vi "Main.vi"(11 "Module Admin":refnum<class "Delacor_lib_QMH_Module Admin.lvclass">) -> ()   [LabVIEW 2021, in "Test Panel GUI Update.lvlib"]
doc: "This template is based off of the Queued Message Handler design pattern and the Queued Message Handler project template that ships with LabVIEW.\n\nThe main difference is that the queue is private to this module and communication between modules is performed via Broadcast and Request events.\n\nRequest events are wrapped in public API methods and are handled in the Event Handling Loop (EHL) of this VI. Any module can register for Broadcast events sent by this module. The EHL generates messages based on user interface actions.\n\nThe Message Handling Loop (MHL) processes messages generated by the EHL, or by other messages. The messages are string values, so new messages can be added easily to the Message Cases case structure in the MHL. Each message cluster can also provide an optional value for Message Data, which is a variant that can be converted to whatever message-specific data is required.\n_____\nBased on DQMH Project Template 7.0.1.1316."
uses:
  Test Panel GUI Update.lvlib
  <vilib>/Delacor/Delacor QMH/Libraries/Module Admin_class/Delacor_lib_QMH_Module Admin.lvclass
  Module Data--cluster.ctl
  Test Panel/GUI Ctrl Data's--Cluster.ctl
  Test Panel/Rx-Mapping Data.ctl
  Capsule-Data's.ctl
  Host-Control's/DIO Data's from RT.ctl
  Host-Control's/AI-Data from RT.ctl
  <vilib>/Wovalab/Utilities/Helper Loop Periodic Timing/Helper Loop Periodic Timing.lvclass/Helper Loop Periodic Timing.ctl
  <vilib>/Delacor/Delacor QMH/Libraries/Message Queue_class/Delacor_lib_QMH_Message Queue.lvclass/Delacor_lib_QMH_Message Queue.ctl
  Host-Control's/Module ID Action Enum.ctl
  RT-Encode Data.ctl
  Stop Argument--cluster.ctl
  <vilib>/Delacor/Delacor QMH/Libraries/Module Admin_class/Delacor_lib_QMH_Module Admin.lvclass/Delacor_lib_QMH_Module Admin.ctl
  Get GUI Ctrl Data Argument--cluster.ctl
  Get GUI Mapping Data's Argument--cluster.ctl
  <vilib>/Utility/miscctls.llb/LVPointTypeDef.ctl
  <vilib>/Delacor/Delacor QMH/Libraries/Message Queue_class/Delacor_lib_QMH_Enqueue Message (Single).vi
  <vilib>/Delacor/Delacor QMH/Libraries/Module Admin_class/Delacor_lib_QMH_Get External Launch.vi
  <vilib>/Wovalab/Utilities/Helper Loop Periodic Timing/U32 Max Value--constant.vi
  <vilib>/Wovalab/Utilities/Helper Loop Periodic Timing/Update Last Execution Time.vi
  <vilib>/Wovalab/Utilities/Helper Loop Periodic Timing/Helper Loop Periodic Timing.lvclass
  <vilib>/Delacor/Delacor QMH/Libraries/Message Queue_class/Delacor_lib_QMH_Message Queue.lvclass
  Test Panel/Test Panel.lvlib
  RT Acquisition Engine/RT Acquisition Engine.lvlib
panel:
  out "error out":errorcluster
  out "Status":string
  in  "Simulate MHL Error":bool
  in  "Simulate EHL Error":bool
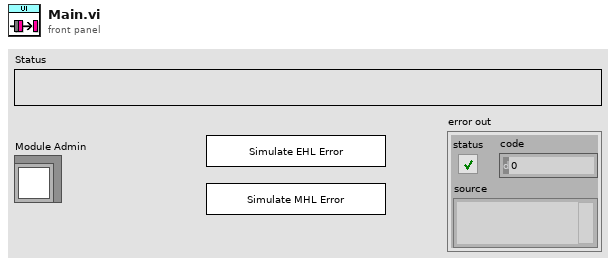
[diagram p1: front panel]
types:
  T1 = typedef "Test Panel GUI Update.lvlib/Request Events--cluster.ctl" = cluster{"Stop Module":refnum<user-event>, "Show Panel":refnum<user-event>, "Hide Panel":refnum<user-event>, "Get Module Execution Status":refnum<user-event>, "Show Diagram":refnum<user-event>, "Get GUI Ctrl Data":refnum<user-event>, "Get GUI Mapping Data's":refnum<user-event>}
  T2 = typedef "Test Panel GUI Update.lvlib/Module Data--cluster.ctl" = cluster{"Status":string, "GUI Ctrl Data's":T3, "Rx-Mapping Data":T4, "Capsule-Data's":T5, "AI Data's":map{string, dbl}}
  T3 = typedef "Test Panel.lvlib/GUI Ctrl Data's--Cluster.ctl" = cluster{"All Ctrl and Indi Label":string[], "All Ctrl & Indi Ref":refnum<vi>[]}
  T4 = typedef "Test Panel.lvlib/Rx-Mapping Data.ctl" = cluster{"Mapped Ctrl and Indi Label":string[], "Mapped Hardware Name":string[], "Mapped Interface Name":string[], "Mapped Channel Name":string[]}
  T5 = typedef "Test Panel GUI Update.lvlib/Capsule-Data's.ctl" = cluster{"DIO Data's":T6, "AI-Info":T7}
  T6 = typedef "DIO Data's from RT.ctl" = cluster{"Channels":string[], "Data":bool[], "Time":string}
  T7 = typedef "AI-Data from RT.ctl" = cluster{"Channel Name's":string[], "Channel Data's":dbl[], "Date & Time":string}
  T8 = typedef "Test Panel GUI Update.lvlib/RT-Encode Data.ctl" = cluster{"Hardware Name":string, "Interface Name":string, "Data":variant}
  T9 = typedef "Module ID Action Enum.ctl" = enum16{"Init", "Insert", "Get a ID", "Get all ID"}
  T10 = enum32{"invalid lock state", "Not Locked", "Locked (No Password)", "Password-protected"}
  T11 = typedef "Test Panel GUI Update.lvlib/Stop Argument--cluster.ctl" = cluster{"Origin":string, "Exit via Stop Module Req?":bool, "Wait for Module to stop?":bool}
  T12 = typedef "Test Panel GUI Update.lvlib/Get GUI Ctrl Data Argument--cluster.ctl" = cluster{"GUI Ctrl Data's":variant}
  T13 = typedef "Test Panel GUI Update.lvlib/Get GUI Mapping Data's Argument--cluster.ctl" = cluster{"Mapping Deatils":variant}
  T14 = typedef "LVPointTypeDef.ctl" = cluster{"Horizontal":i16, "Vertical":i16}
  T15 = enum32{"Invalid", "Standard", "Closed", "Hidden", "Minimized", "Maximized"}
  T16 = typedef "RT Acquisition Engine.lvlib/Broadcast Events--cluster.ctl" = cluster{"Module Did Init":refnum<user-event>, "Status Updated":refnum<user-event>, "Error Reported":refnum<user-event>, "Module Did Stop":refnum<user-event>, "Update Module Execution Status":refnum<user-event>, "RT Connection Status":refnum<user-event>, "Tx RT Hardware Info":refnum<user-event>, "DO Data's":refnum<user-event>, "AI-Info":refnum<user-event>}
  T17 = typedef "HW Name Enum.ctl" = enum16{"Capsule-1", "Capsule-2", "Capsule-3", "Capsule-4", "sb-RIO", "Safety", "Release"}
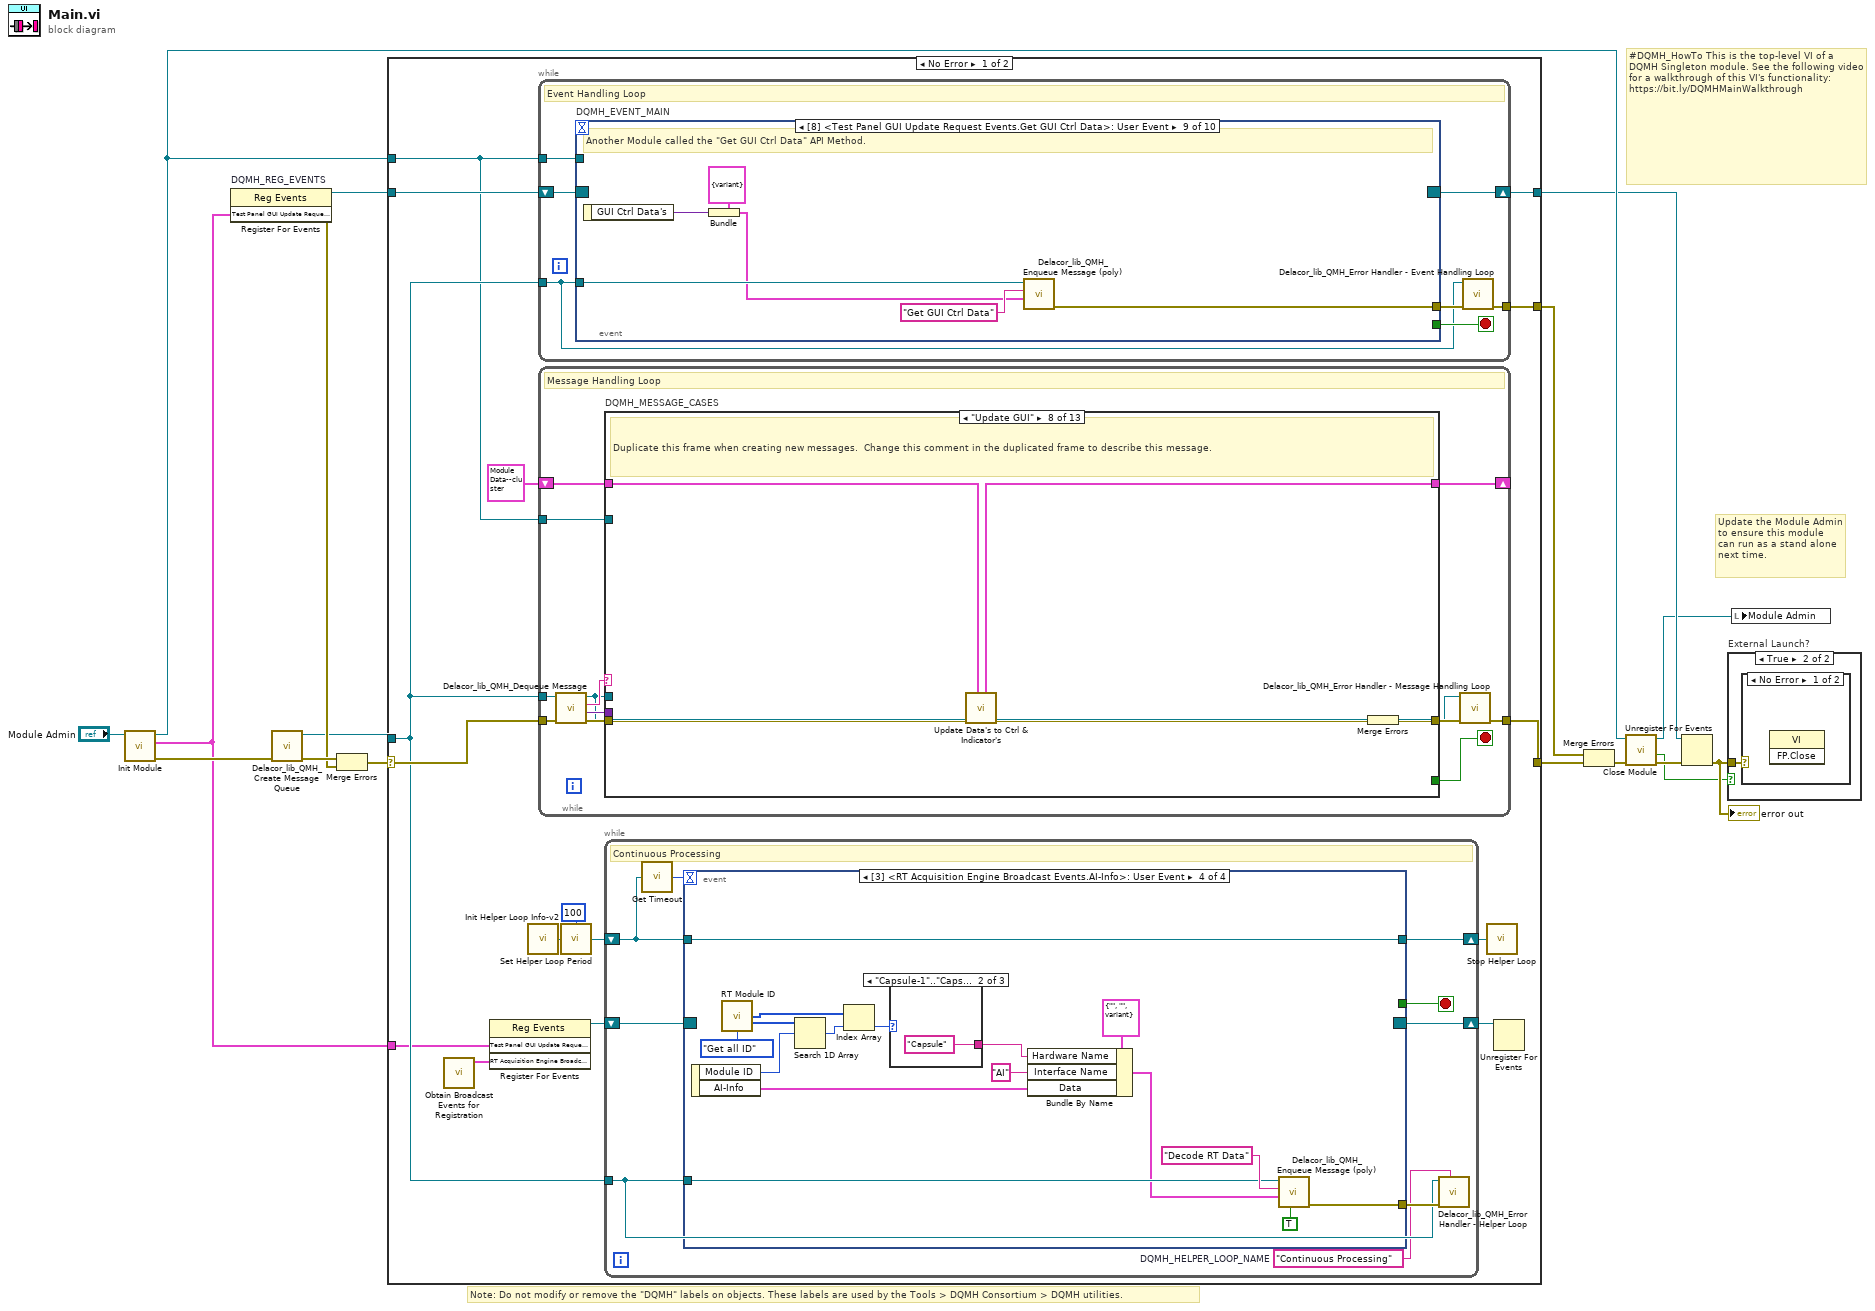
[diagram p0: block diagram]
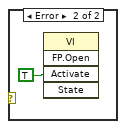
[diagram p3: hidden frame]
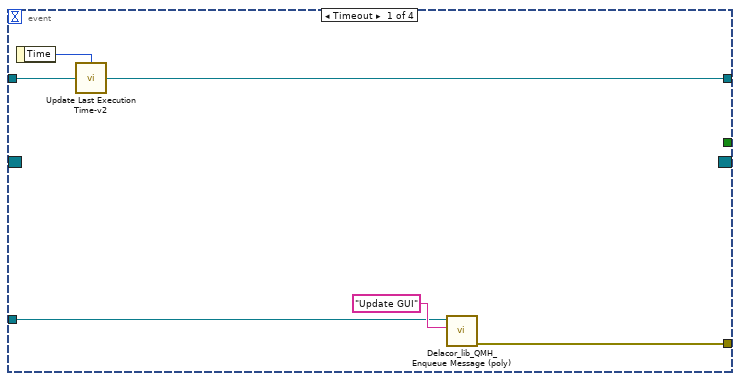
[diagram p4: hidden frame]
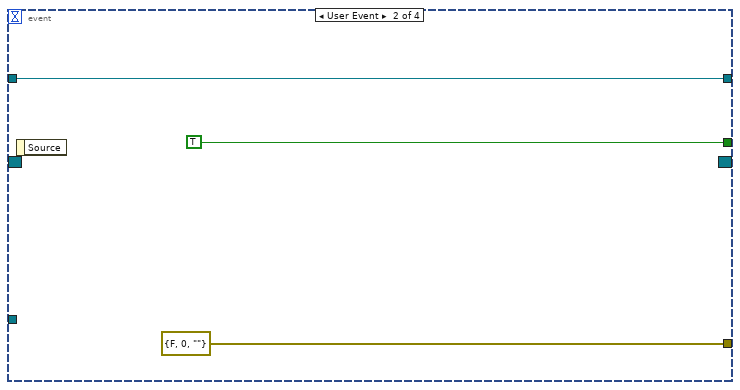
[diagram p5: hidden frame]
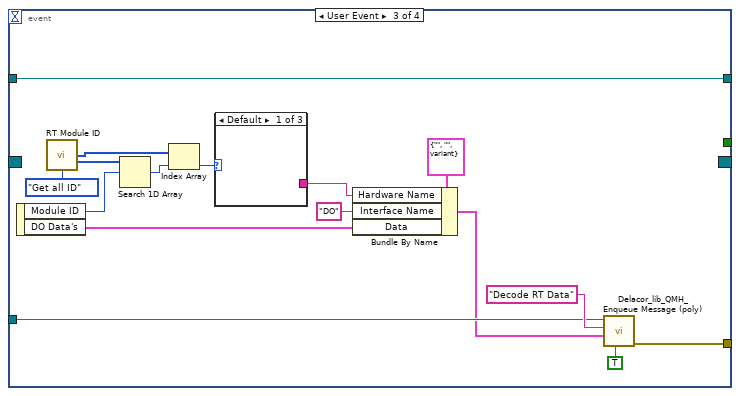
[diagram p6: hidden frame]
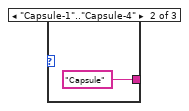
[diagram p7: hidden frame]
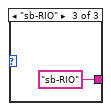
[diagram p8: hidden frame]
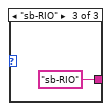
[diagram p10: hidden frame]
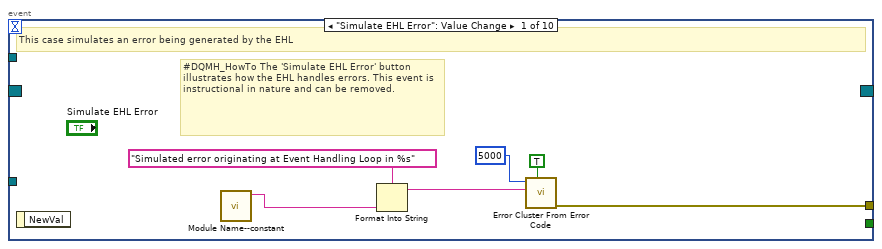
[diagram p11: hidden frame]
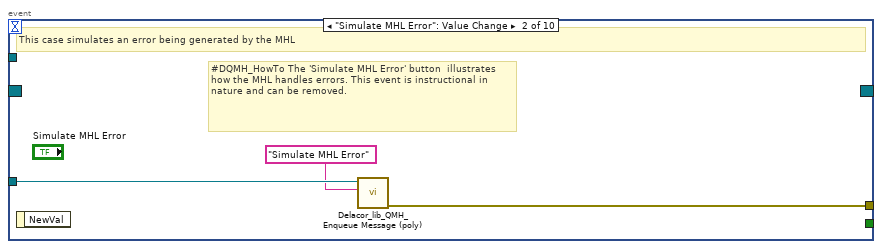
[diagram p12: hidden frame]
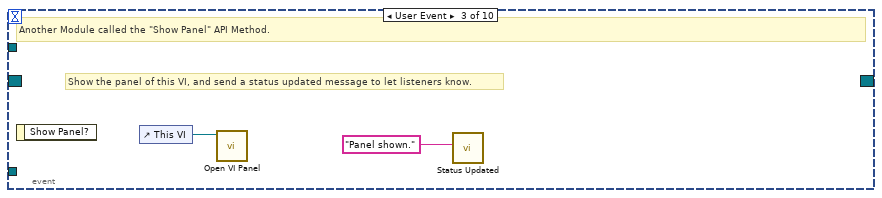
[diagram p13: hidden frame]
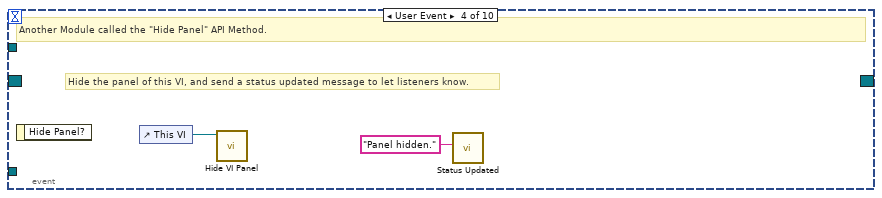
[diagram p14: hidden frame]
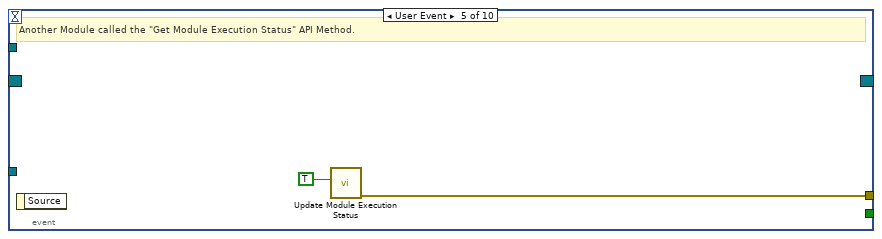
[diagram p15: hidden frame]
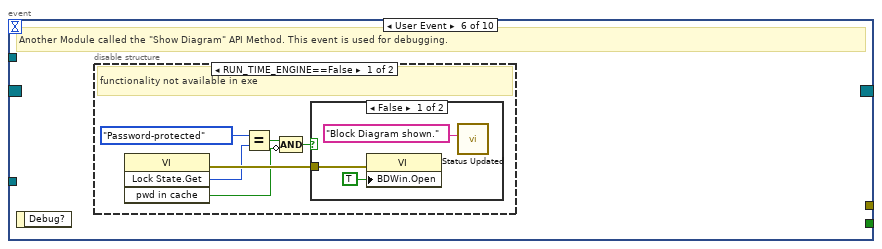
[diagram p16: hidden frame]
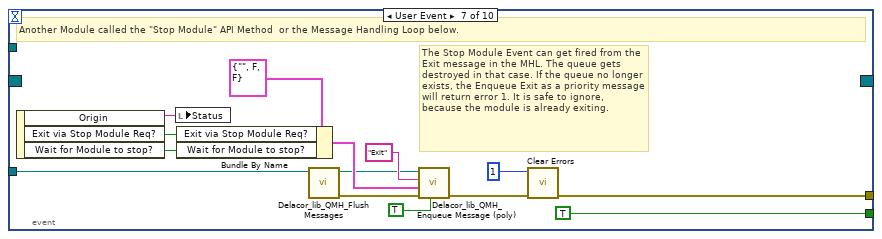
[diagram p19: hidden frame]
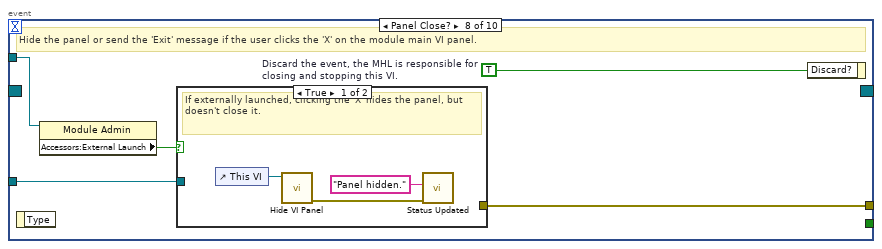
[diagram p20: hidden frame]
diagram:
  # "#DQMH_HowTo This is the top-level VI of a DQMH Singleton module. See the following video for a walkthrough of this VI's functionality: https://bit.ly/DQMHMainWalkthrough"
  # "Note: Do not modify or remove the \"DQMH\" labels on objects. These labels are used by the Tools > DQMH Consortium > DQMH utilities."
  # "Update the Module Admin to ensure this module can run as a stand alone next time."
  n1 = call "Init Module.vi"("Singleton Module Admin in"="Module Admin") -> ("error out"=w16:errorcluster, "Test Panel GUI Update Request Events"=w1:T1, "Singleton Module Admin out"=w8:refnum<class "Delacor_lib_QMH_Module Admin.lvclass">)  [unwired: 8 in]
  n2 = register-events "DQMH_REG_EVENTS"(w1) -> (reference out=w6:refnum<event-registration>, error out=w9:errorcluster)  [unwired: 2 in]
  n3 = call <vilib>:"Delacor_lib_QMH_Create Message Queue.vi"("error in"=w16) -> ("error out"=w11:errorcluster, "Message Queue"=w5:refnum<class "Delacor_lib_QMH_Message Queue.lvclass">)  [unwired: 9 in]
  n4 = Merge Errors(w11, w9) -> (w10:errorcluster)
  n5 = case shown="No Error" w10 {
    selector: w10 -> [w31 w296]
    tunnel: [w33 w295] -> w17
    tunnel: [w30 w294] -> w7
    tunnel: w6 -> [w28 w294]
    tunnel: w5 -> [w27 w289]
    tunnel: [w32 _] -> w14
    tunnel: w8 -> [w26 w290]
    tunnel: w1 -> [w25 _]
    frame No Error {
      n6 = call "Obtain Broadcast Events for Registration.vi"() -> ("RT Acquisition Engine Broadcast Events"=w18:T16)  [unwired: 9 in, 2 out]
      n7 = register-events ("DQMH_HELPER_REGFOREVENTS")(w25, w18) -> (reference out=w23:refnum<event-registration>)  [unwired: 2 in, 1 out]
      n8 = call <vilib>:"Init Helper Loop Info-v2.vi"() -> ("Helper Loop Periodic Timing"=w20:refnum<class "Helper Loop Periodic Timing.lvclass">)  [unwired: 1 in]
      n9 = while {
        tunnel: w27 -> [w88]
        shift-right: [w91] -> w30
        shift-left: w28 -> [w92]
        tunnel: [w93] -> w32
        tunnel: w26 -> [w89]
        stop <- w90 stop-if-true
        # "Event Handling Loop"
        n10 = event "DQMH_EVENT_MAIN" shown="[8] <Test Panel GUI Update Request Events.Get GUI Ctrl Data>: User Event" {
          selector: w92 -> [_ _ _ _ _ _ _ _ _ _]
          dyn-events: [_ _ _ _ _ _ _ _ _ _] -> w91
          timeout: _ -> [_ _ _ _ _ _ _ _ _ _]
          tunnel: [_ _ _ _ _ _ TRUE ("Discard?") _ _ _] -> w90
          tunnel: w88 -> [_ w102 _ _ _ _ w121 w135 w150 w156]
          tunnel: [w100 w103 _ _ w109 _ w131 w137 w145 w151] -> w94
          tunnel: w89 -> [_ _ _ _ _ _ _ w134 _ _]
          event "Simulate EHL Error": Value Change {
            # "#DQMH_HowTo The 'Simulate EHL Error' button  illustrates how the EHL handles errors. This event is instructional in nature and can be removed."
            # "This case simulates an error being generated by the EHL"
            n11 = event-data() -> ()  [unwired: 1 in, 1 out]
            n12 = call "Module Name--constant.vi"() -> ("Module Name"=w97:string)  [unwired: 11 in]
            n13 = Format Into String(format string="Simulated error originating at Event Handling Loop in %s", w97) -> (resulting string=w98:string)  [unwired: 2 in, 1 out]
            n14 = call <vilib>:"Error Cluster From Error Code.vi"("show call chain? (False)"=TRUE, "error message (\"\")"=w98, "error code (0)"=5000) -> ("error out"=w100:errorcluster)  [unwired: 6 in]
          }
          event "Simulate MHL Error": Value Change {
            # "#DQMH_HowTo The 'Simulate MHL Error' button  illustrates how the MHL handles errors. This event is instructional in nature and can be removed."
            # "This case simulates an error being generated by the MHL"
            n15 = event-data() -> ()  [unwired: 1 in, 1 out]
            n16 = call-poly <vilib>:"Delacor_lib_QMH_Enqueue Message (poly).vi"("Message"="Simulate MHL Error", "Message Queue in"=w102) -> ("error out"=w103:errorcluster)  [unwired: 8 in, 1 out]
          }
          event User Event {
            # "Show the panel of this VI, and send a status updated message to let listeners know."
            # "Another Module called the \"Show Panel\" API Method."
            n17 = event-data() -> ()  [unwired: 1 in, 1 out]
            n18 = control-ref of="This VI"() -> (w105:refnum<vi>)
            n19 = call "Open VI Panel.vi"("VI"=w105) -> ()  [unwired: 10 in, 1 out]
            n20 = call "Status Updated.vi"("Status"="Panel shown." ("format string")) -> ()  [unwired: 10 in, 1 out]
          }
          event User Event {
            # "Hide the panel of this VI, and send a status updated message to let listeners know."
            # "Another Module called the \"Hide Panel\" API Method."
            n21 = event-data() -> ()  [unwired: 1 in, 1 out]
            n22 = control-ref of="This VI"() -> (w107:refnum<vi>)
            n23 = call "Hide VI Panel.vi"("VI"=w107) -> ()  [unwired: 10 in, 1 out]
            n24 = call "Status Updated.vi"("Status"="Panel hidden." ("format string")) -> ()  [unwired: 10 in, 1 out]
          }
          event User Event {
            # "Another Module called the \"Get Module Execution Status\" API Method."
            n25 = event-data() -> ()  [unwired: 1 in, 1 out]
            n26 = call "Update Module Execution Status.vi"("Running?"=TRUE) -> ("error out"=w109:errorcluster)  [unwired: 10 in]
          }
          event User Event {
            # "Another Module called the \"Show Diagram\" API Method. This event is used for debugging."
            n27 = event-data() -> ()  [unwired: 1 in, 1 out]
            n28 = disable-structure shown="RUN_TIME_ENGINE==False" {
              frame condition #0 (active) {
                # "functionality not available in exe"
                n29 = invoke on="Invoke Node" class="VI" method="Lock State.Get"() -> (error out=w115:errorcluster, "Get Lock State"=w114:T10, "pwd in cache"=w111:bool)  [unwired: 4 in, 1 out]
                n30 = Equal?(x=T10."Password-protected", y=w114) -> (x = y?=w112:bool)
                n31 = Compound Arithmetic op=AND(w112, invert w111) -> (w110:bool)
                n32 = case shown="False" w110 {
                  tunnel: w115 -> [w118 _]
                  frame False {
                    n33 = property on="Property Node" class="VI"(error in=w118, "BDWin.Open"=TRUE ("Block Diagram Window:Open")) -> ()  [unwired: 1 in, 2 out]
                    n34 = call "Status Updated.vi"("Status"="Block Diagram shown." ("format string")) -> ()  [unwired: 10 in, 1 out]
                  }
                  frame True {
                    # "Password-protected VI, and the password is not in the cache. Do not show the diagram."
                  }
                }
              }
              frame condition #1 {
              }
            }
          }
          event User Event {
            # "The Stop Module Event can get fired from the Exit message in the MHL. The queue gets destroyed in that case. If the queue no longer exists, the Enqueue Exit as a priority message will return error 1. It is safe to ignore, because the module is already exiting."
            # "Another Module called the \"Stop Module\" API Method  or the Message Handling Loop below."
            n35 = event-data() -> ("Origin"=w128:string, "Exit via Stop Module Req?"=w124:bool, "Wait for Module to stop?"=w123:bool)  [unwired: 1 in]
            n36 = local write "Status"(w128) -> ()
            n37 = Bundle By Name(cluster=T11 {"Origin"="", "Exit via Stop Module Req?"=FALSE, "Wait for Module to stop?"=FALSE} ("Stop Argument"), "Exit via Stop Module Req?"=w124, "Wait for Module to stop?"=w123) -> (w122:T11)
            n38 = call-dynamic "Delacor_lib_QMH_Flush Messages.vi"("Message Queue in"=w121) -> ("error out"=w119:errorcluster, "Message Queue out"=w120:refnum<class "Delacor_lib_QMH_Message Queue.lvclass">)  [unwired: 7 in, 2 out]
            n39 = call-poly <vilib>:"Delacor_lib_QMH_Enqueue Message (poly).vi"("Priority Message? (F)"=TRUE, "error in"=w119, "Message Data"=w122, "Message"="Exit", "Message Queue in"=w120) -> ("error out"=w132:errorcluster)  [unwired: 5 in, 1 out]
            n40 = call <vilib>:"Clear Errors.vi"("error in (no error)"=w132, "specific error code to clear (0: all)"=1) -> ("error out"=w131:errorcluster)  [unwired: 4 in, 1 out]
          }
          event Panel Close? {
            w136 = TRUE  # Discard the event, the MHL is responsible for closing and stopping this VI.
            # "Hide the panel or send the 'Exit' message if the user clicks the 'X' on the module main VI panel."
            n41 = event-data() -> ()  [unwired: 1 in, 1 out]
            n42 = property on="Property Node" class="Module Admin"(reference=w134) -> ("Accessors:External Launch"=w133:bool)  [unwired: 1 in, 2 out]
            n43 = case shown="True" w133 {
              tunnel: w135 -> [_ w143]
              tunnel: [_ w144] -> w137
              frame True {
                # "If externally launched, clicking the 'X' hides the panel, but doesn't close it."
                n44 = control-ref of="This VI"() -> (w140:refnum<vi>)
                n45 = call "Hide VI Panel.vi"("VI"=w140) -> ("error out"=w138:errorcluster)  [unwired: 10 in]
                n46 = call "Status Updated.vi"("error in"=w138, "Status"="Panel hidden." ("format string")) -> ()  [unwired: 9 in, 1 out]
              }
              frame False {
                # "If run as a stand-alone VI, clicking the panel 'X' stops the VI."
                n47 = call-poly <vilib>:"Delacor_lib_QMH_Enqueue Message (poly).vi"("Priority Message? (F)"=TRUE, "Message"="Exit", "Message Queue in"=w143) -> ("error out"=w144:errorcluster)  [unwired: 7 in, 1 out]
              }
            }
            n48 = event-data ("Event Filter Node")("Discard?"=w136) -> ()  [unwired: 1 in, 1 out]
          }
          event User Event {
            # "Another Module called the \"Get GUI Ctrl Data\" API Method."
            n49 = event-data() -> ("GUI Ctrl Data's"=w146:variant)  [unwired: 1 in]
            n50 = Bundle(cluster=T12 {"GUI Ctrl Data's"=variant} ("Get GUI Ctrl Data Argument"), "GUI Ctrl Data's"=w146) -> (w147:T12)
            n51 = call-poly <vilib>:"Delacor_lib_QMH_Enqueue Message (poly).vi"("Message Data"=w147, "Message"="Get GUI Ctrl Data", "Message Queue in"=w150) -> ("error out"=w145:errorcluster)  [unwired: 7 in, 1 out]
          }
          event User Event {
            # "Another Module called the \"Get GUI Mapping Data's\" API Method."
            n52 = event-data() -> ("Mapping Deatils"=w152:variant)  [unwired: 1 in]
            n53 = Bundle(cluster=T13 {"Mapping Deatils"=variant} ("Get GUI Mapping Data's Argument"), "Mapping Deatils"=w152) -> (w153:T13)
            n54 = call-poly <vilib>:"Delacor_lib_QMH_Enqueue Message (poly).vi"("Message Data"=w153, "Message"="Get GUI Mapping Data's", "Message Queue in"=w156) -> ("error out"=w151:errorcluster)  [unwired: 7 in, 1 out]
          }
        }
        n55 = call-dynamic "Delacor_lib_QMH_Error Handler - Event Handling Loop.vi"("error in"=w94, "Message Queue in"=w88) -> ("dup error in"=w93:errorcluster)  [unwired: 8 in, 1 out]
      }
      n56 = while {
        tunnel: w27 -> [w157]
        shift-right: [w165] -> _
        shift-left: T2 {"Status"="", "GUI Ctrl Data's"={"All Ctrl and Indi Label"=[], "All Ctrl & Indi Ref"=[]}, "Rx-Mapping Data"={"Mapped Ctrl and Indi Label"=[], "Mapped Hardware Name"=[], "Mapped Interface Name"=[], "Mapped Channel Name"=[]}, "Capsule-Data's"={"DIO Data's"={"Channels"=[], "Data"=[], "Time"=""}, "AI-Info"={"Channel Name's"=[], "Channel Data's"=[], "Date & Time"=""}}, "AI Data's"={}} ("Data Cluster") -> [w166]
        tunnel: w31 -> [w168]
        tunnel: [w160] -> w33
        tunnel: w26 -> [w161]
        stop <- w164 stop-if-true
        # "Message Handling Loop"
        n57 = call-dynamic "Delacor_lib_QMH_Dequeue Message.vi"("error in"=w168, "Message Queue in"=w157) -> ("error out"=w167:errorcluster, "Message Data"=w162:variant, "Message"=w163:string, "Message Queue out"=w158:refnum<class "Delacor_lib_QMH_Message Queue.lvclass">)  [unwired: 6 in]
        n58 = case "DQMH_MESSAGE_CASES" shown="\"Update GUI\"" w163 {
          selector: w163 -> [_ _ _ _ _ _ _ _ _ _ _ _ w284]
          tunnel: w158 -> [_ _ _ _ _ w221 _ _ _ _ w250 w272 _]
          tunnel: w167 -> [w186 w190 w201 w212 w215 w225 w228 w234 w237 w246 w257 w278 w287]
          tunnel: [w184 w190 w196 w206 w214 w227 w230 w235 w237 w245 w253 w273 w288] -> w159
          tunnel: w166 -> [w175 w189 w193 w205 w213 w216 w229 w232 w236 w243 w252 w271 w285]
          tunnel: [w174 w189 w192 w204 w213 w217 w229 w231 w236 w243 w252 w271 w285] -> w165
          tunnel: [_ _ _ _ _ _ _ _ _ _ _ w270 _] -> w164
          tunnel: w162 -> [_ _ w200 w211 _ w226 _ _ _ _ w251 w269 _]
          tunnel: w161 -> [w176 _ _ _ _ _ _ _ _ _ w249 w264 _]
          frame "Initialize" {
            w170 = "Initial Message" ("Initial Message")
            # "#CodeNeeded - Initialize the appearance of the front panel."
            # "#CodeNeeded - Initialize your state data here."
            # "Initialize - Any operation that needs to be done before the module can receive messages. Synchronize Caller Events.vi will inform Start Module.vi that the module has launched and is ready to receive messages. Module Did Init.vi will broadcast that the module initialized."
            n59 = call "Synchronize Caller Events.vi"("error in"=w186, "Singleton Module Admin in"=w176) -> ("error out"=w185:errorcluster, "Singleton Module Admin out"=w171:refnum<class "Delacor_lib_QMH_Module Admin.lvclass">)  [unwired: 8 in]
            n60 = property on="Property Node" class="Module Admin"(reference=w171) -> ("Accessors:External Launch"=w180:bool)  [unwired: 1 in, 2 out]
            n61 = Select(t=T15."Hidden" ("State"), s=w180, f=T15."Standard" ("State")) -> (s? t:f=w177:T15)
            n62 = call "Module Name--constant.vi"() -> ("Module Name"=w183:string)  [unwired: 11 in]
            n63 = property on="Property Node" class="VI"("Front Panel.Title"=w183) -> (reference out=w182:refnum<vi>, error out=w188:errorcluster)  [unwired: 2 in]
            n64 = call "Module Name--constant.vi"() -> ("Module Name"=w172:string)  [unwired: 11 in]
            n65 = invoke on="Invoke Node" class="VI" method="FP.Open"(reference=w182, error in=w188, "State"=w177) -> (reference out=w181:refnum<vi>, error out=w187:errorcluster)  [unwired: 2 in, 3 out]
            n66 = Bundle By Name(cluster=w175, "Status"=w170) -> (w174:T2)
            n67 = call "Module Did Init.vi"("error in"=w185, "Initialized?"=TRUE, "Origin"=w172) -> ("error out"=w184:errorcluster)  [unwired: 8 in]
            n68 = invoke on="Invoke Node" class="VI" method="FP.Center"(reference=w181, error in=w187) -> ()  [unwired: 1 in, 3 out]
            n69 = property on="Pane" class="Pane"("Origin"=T14 {"Horizontal"=0, "Vertical"=0}) -> ()  [unwired: 2 in, 2 out]
            "Status" <- w170
          }
          frame "---Module Specific---" {
            # "Separator -- The following cases handle messages specific to this Module."
          }
          frame "Get GUI Ctrl Data" {
            # "This Event will request the GUI Ctrl Data's from the Test Panel Module."
            n70 = Variant To Data(error in=w201, type=T12 {"GUI Ctrl Data's"=variant} ("Get GUI Ctrl Data Argument"), Variant=w200) -> (data=w198:T12, error out=w197:errorcluster)
            n71 = Unbundle By Name(w198) -> ("GUI Ctrl Data's"=w195:variant)
            n72 = Variant To Data(error in=w197, type=T3 {"All Ctrl and Indi Label"=[], "All Ctrl & Indi Ref"=[]} ("GUI Ctrl Data's"), Variant=w195) -> (data=w191:T3, error out=w196:errorcluster)
            n73 = Bundle By Name(cluster=w193, "GUI Ctrl Data's"=w191) -> (w192:T2)
          }
          frame "Get GUI Mapping Data's" {
            # "This Request Event will give the Mapping details for the controll's and indicator's present in the Test Panel Module."
            n74 = Variant To Data(error in=w212, type=T13 {"Mapping Deatils"=variant} ("Get GUI Mapping Data's Argument"), Variant=w211) -> (data=w209:T13, error out=w207:errorcluster)
            n75 = Unbundle By Name(w209) -> ("Mapping Deatils"=w208:variant)
            n76 = Variant To Data(error in=w207, type=T4 {"Mapped Ctrl and Indi Label"=[], "Mapped Hardware Name"=[], "Mapped Interface Name"=[], "Mapped Channel Name"=[]} ("Rx-Mapping Data"), Variant=w208) -> (data=w203:T4, error out=w206:errorcluster)
            n77 = Bundle By Name(cluster=w205, "Rx-Mapping Data"=w203) -> (w204:T2)
          }
          frame "---Copy This Frame---" {
            # "Duplicate this frame when creating new messages.  Change this comment in the duplicated frame to describe this message."
            n78 = Merge Errors(w215) -> (w214:errorcluster)
          }
          frame "Decode RT Data" {
            # "Duplicate this frame when creating new messages.  Change this comment in the duplicated frame to describe this message."
            n79 = Variant To Data(error in=w225, type=T8 {"Hardware Name"="", "Interface Name"="", "Data"=variant} ("RT-Decode Data"), Variant=w226) -> (data=w220:T8, error out=w219:errorcluster)
            n80 = call "Seperate Channel Data's.vi"("Data Cluster In"=w216, "error In"=w219, "RT-Decode Data"=w220) -> ("error out"=w218:errorcluster, "Data Cluster Out"=w217:T2)  [unwired: 7 in]
            n81 = call-poly <vilib>:"Delacor_lib_QMH_Enqueue Message (poly).vi"("error in"=w218, "Message"="Update GUI", "Message Queue in"=w221) -> ("error out"=w222:errorcluster)  [unwired: 7 in, 1 out]
            n82 = Merge Errors(w222) -> (w227:errorcluster)
          }
          frame "Upate Data" {
            # "Duplicate this frame when creating new messages.  Change this comment in the duplicated frame to describe this message."
            n83 = Merge Errors(w228) -> (w230:errorcluster)
          }
          frame "Update GUI" {
            # "Duplicate this frame when creating new messages.  Change this comment in the duplicated frame to describe this message."
            n84 = call "Update Data's to Ctrl & Indicator's.vi"("Data Cluster In"=w232, "error in (no error)"=w234) -> ("error out"=w233:errorcluster, "Data Cluster Out"=w231:T2)  [unwired: 8 in]
            n85 = Merge Errors(w233) -> (w235:errorcluster)
          }
          frame "---Exit and Error Handling---" {
            # "Separator - The following cases handle errors and exit messages."
          }
          frame "Simulate MHL Error" {
            # "#DQMH_HowTo The 'Simulate MHL Error' button  illustrates how the MHL handles errors. This event is instructional in nature and can be removed."
            # "Simulate an error occurring at the MHL"
            n86 = call "Module Name--constant.vi"() -> ("Module Name"=w239:string)  [unwired: 11 in]
            n87 = Format Into String(format string="Simulated error originating at Message Handling Loop in %s", w239) -> (resulting string=w240:string)  [unwired: 2 in, 1 out]
            n88 = call <vilib>:"Error Cluster From Error Code.vi"("show call chain? (False)"=TRUE, "error message (\"\")"=w240, "error code (0)"=5001) -> ("error out"=w244:errorcluster)  [unwired: 6 in]
            n89 = Merge Errors(w246, w244) -> (w245:errorcluster)
          }
          frame "Error" {
            # "#CodeRecommended - If the module is running in standalone mode (External Launch = FALSE), this code will pop up an error dialog and call the 'Exit' message if an error occurs. Add more fine-grained error management here."
            # "Error - Check the error message data and respond accordingly. This message is sent by the \"Error Handler\" VIs at the end of each loop in this application."
            n90 = property on="Property Node" class="Module Admin"(reference=w249) -> ("Accessors:External Launch"=w248:bool)  [unwired: 1 in, 2 out]
            n91 = Variant To Data(error in=w257, type=errorcluster {"status"=FALSE, "code"=0, "source"=""} ("error constant"), Variant=w251) -> (data=w247:errorcluster, error out=w255:errorcluster)
            n92 = local write "error out"(w247) -> ()
            n93 = call "Error Reported.vi"("Error"=w247) -> ()  [unwired: 10 in, 1 out]
            n94 = case shown="False" w248 {
              tunnel: [w262 _] -> w254
              tunnel: w250 -> [w260 _]
              tunnel: w247 -> [w261 _]
              frame False {
                n95 = disable-structure shown="Default" {
                  disable-tunnel: w261 -> [w263 _]
                  frame condition #0 (active) {
                    # "If the module is running standalone, then pop up an error dialog and call the \"Exit\" message."
                    n96 = call <vilib>:"Simple Error Handler.vi"("error in (no error)"=w263) -> ()  [unwired: 4 in, 5 out]
                  }
                  frame condition #1 {
                    # "To prevent the Simple Error Handler VI from being loaded (e.g. when deploying to a Real-Time target), add the Conditional Disable Symbol \"DQMH_Disable_SEH\" to your project and set it to TRUE."
                  }
                }
                n97 = call-poly <vilib>:"Delacor_lib_QMH_Enqueue Message (poly).vi"("Priority Message? (F)"=TRUE, "Message"="Exit", "Message Queue in"=w260) -> ("error out"=w262:errorcluster)  [unwired: 7 in, 1 out]
              }
              frame True {
                # "If the module was launched externally, calling the Error Reported broadcast VI is the only action performed by the \"Error\" message. The module's caller can then process the error appropriately."
              }
            }
            n98 = Merge Errors(w255, w254) -> (w253:errorcluster)
          }
          frame "Exit" {
            w268 = 91  # 91: not all Exit messages will have an argument
            w270 = TRUE  # Stop the VI
            # "Release the message queue reference"
            # "#CodeNeeded - Add any required cleanup code here."
            # "Exit - Exit the application."
            n99 = Variant To Data(error in=w278, type=T11 {"Origin"="", "Exit via Stop Module Req?"=FALSE, "Wait for Module to stop?"=FALSE} ("Stop Argument"), Variant=w269) -> (data=w266:T11, error out=w275:errorcluster)
            n100 = call <vilib>:"Clear Errors.vi"("error in (no error)"=w275, "specific error code to clear (0: all)"=w268) -> ("error out"=w277:errorcluster)  [unwired: 4 in, 1 out]
            n101 = control-ref of="This VI"() -> (w265:refnum<vi>)
            n102 = call-dynamic "Delacor_lib_QMH_Release Message Queue.vi"("error in"=w277, "Message Queue"=w272) -> ("error out"=w276:errorcluster)  [unwired: 9 in]
            n103 = call "Handle Exit.vi"("Stop Argument"=w266, "Admin in"=w264, "VI reference"=w265) -> ("error out"=w274:errorcluster)  [unwired: 7 in, 1 out]
            n104 = Merge Errors(w276, w274) -> (w273:errorcluster)
            n105 = call "Error Reported.vi"("Error"=w273) -> ()  [unwired: 10 in, 1 out]
          }
          frame Default {
            # "'Default' case only runs if there is a message that isn't defined in any of the other cases.  Output a programming error."
            n106 = call "Module Name--constant.vi"() -> ("Module Name"=w283:string)  [unwired: 11 in]
            n107 = Format Into String(format string="The invalid message string \"%s\" was received in the Message Handling Loop for module \"%s\".", w284, w283) -> (resulting string=w279:string)  [unwired: 2 in, 1 out]
            n108 = call <vilib>:"Error Cluster From Error Code.vi"("show call chain? (False)"=TRUE, "error message (\"\")"=w279, "error code (0)"=1) -> ("error out"=w286:errorcluster)  [unwired: 6 in]
            n109 = Merge Errors(w287, w286) -> (w288:errorcluster)
          }
        }
        n110 = call-dynamic "Delacor_lib_QMH_Error Handler - Message Handling Loop.vi"("error in"=w159, "Message Queue in"=w158) -> ("dup error in"=w160:errorcluster)  [unwired: 8 in, 1 out]
      }
      n111 = call <vilib>:"Set Helper Loop Period.vi"("Period (ms)"=100, "Helper Loop Periodic Timing in"=w20) -> ("Helper Loop Periodic Timing out"=w21:refnum<class "Helper Loop Periodic Timing.lvclass">)  [unwired: 13 in]
      n112 = while "DQMH_HELPER_LOOP" {
        shift-right: [w42] -> w19
        shift-left: w21 -> [w34]
        shift-right: [w40] -> w24
        shift-left: w23 -> [w41]
        tunnel: w27 -> [w37]
        stop <- w39 stop-if-true
        w36 = "Continuous Processing"  # DQMH_HELPER_LOOP_NAME
        # "Continuous Processing"
        n113 = call <vilib>:"Get Timeout.vi"("Helper Loop Periodic Timing"=w34) -> ("Timeout (ms)"=w35:i32)  [unwired: 12 in, 2 out]
        n114 = event "DQMH_HELPER_EVENT_STRUCTURE" shown="[3] <RT Acquisition Engine Broadcast Events.AI-Info>: User Event" {
          selector: w41 -> [_ _ _ _]
          dyn-events: [_ _ _ _] -> w40
          timeout: w35 -> [_ _ _ _]
          tunnel: w34 -> [w47 w51 w67 w85]
          tunnel: [w46 w51 w67 w85] -> w42
          tunnel: [_ TRUE _ _] -> w39
          tunnel: [w43 errorcluster {"status"=FALSE, "code"=0, "source"=""} ("error constant") w55 w74] -> w38
          tunnel: w37 -> [w44 _ w54 w73]
          event Timeout {
            n115 = event-data() -> ("Time"=w48:u32)  [unwired: 1 in]
            n116 = call <vilib>:"Update Last Execution Time-v2.vi"("Time"=w48, "Helper Loop Periodic Timing in"=w47) -> ("Helper Loop Periodic Timing out"=w46:refnum<class "Helper Loop Periodic Timing.lvclass">)  [unwired: 12 in, 1 out]
            n117 = call-poly <vilib>:"Delacor_lib_QMH_Enqueue Message (poly).vi"("Message"="Update GUI", "Message Queue in"=w44) -> ("error out"=w43:errorcluster)  [unwired: 8 in, 1 out]
          }
          event User Event {
            n118 = event-data() -> ()  [unwired: 1 in, 1 out]
          }
          event User Event {
            n119 = event-data() -> ("Module ID"=w62:i32, "DO Data's"=w57:T6)  [unwired: 1 in]
            n120 = call "RT Module ID.vi"("Action"=Module_ID_Action_Enum."Get all ID") -> ("All HW Name Out"=w63:T17[], "All HW-ID Out"=w64:i32[])  [unwired: 11 in, 2 out]
            n121 = Search 1D Array(1D array=w64, element=w62) -> (index of element=w65:i32)  [unwired: 1 in]
            n122 = Index Array(array=w63, index=w65) -> (element=w61:T17)
            n123 = case shown="Default" w61 {
              tunnel: [_ "Capsule" "sb-RIO"] -> w59
              frame Default {
              }
              frame "Capsule-1".."Capsule-4" {
              }
              frame "sb-RIO" {
              }
            }
            n124 = Bundle By Name(cluster=T8 {"Hardware Name"="", "Interface Name"="", "Data"=variant} ("RT-Decode Data"), "Hardware Name"=w59, "Interface Name"="DO", "Data"=w57) -> (w53:T8)
            n125 = call-poly <vilib>:"Delacor_lib_QMH_Enqueue Message (poly).vi"("Priority Message? (F)"=TRUE, "Message Data"=w53, "Message"="Decode RT Data", "Message Queue in"=w54) -> ("error out"=w55:errorcluster)  [unwired: 6 in, 1 out]
          }
          event User Event {
            n126 = event-data() -> ("Module ID"=w80:i32, "AI-Info"=w70:T7)  [unwired: 1 in]
            n127 = call "RT Module ID.vi"("Action"=Module_ID_Action_Enum."Get all ID") -> ("All HW Name Out"=w81:T17[], "All HW-ID Out"=w82:i32[])  [unwired: 11 in, 2 out]
            n128 = Search 1D Array(1D array=w82, element=w80) -> (index of element=w83:i32)  [unwired: 1 in]
            n129 = Index Array(array=w81, index=w83) -> (element=w79:T17)
            n130 = case shown="\"Capsule-1\"..\"Capsule-4\"" w79 {
              tunnel: [_ "Capsule" "sb-RIO"] -> w77
              frame Default {
              }
              frame "Capsule-1".."Capsule-4" {
              }
              frame "sb-RIO" {
              }
            }
            n131 = Bundle By Name(cluster=T8 {"Hardware Name"="", "Interface Name"="", "Data"=variant} ("RT-Decode Data"), "Hardware Name"=w77, "Interface Name"="AI", "Data"=w70) -> (w72:T8)
            n132 = call-poly <vilib>:"Delacor_lib_QMH_Enqueue Message (poly).vi"("Priority Message? (F)"=TRUE, "Message Data"=w72, "Message"="Decode RT Data", "Message Queue in"=w73) -> ("error out"=w74:errorcluster)  [unwired: 6 in, 1 out]
          }
        }
        n133 = call-dynamic "Delacor_lib_QMH_Error Handler - Helper Loop.vi"("Error Debug"=w36, "error in"=w38, "Message Queue in"=w37) -> ()  [unwired: 7 in, 2 out]
      }
      n134 = call <vilib>:"Stop Helper Loop.vi"("Helper Loop Periodic Timing in"=w19) -> ()  [unwired: 1 out]
      n135 = Unregister For Events(event registration refnum=w24) -> ()  [unwired: 1 in, 1 out]
    }
    frame Error {
      # "Synchronize Caller Events.vi will inform Start Module.vi that the module has launched and will let the code calling Start Module.vi register for broadcasts and would permit the caller receive the broadcast that an error occurred at launch time."
      n136 = call-dynamic "Delacor_lib_QMH_Release Message Queue.vi"("error in"=w296, "Message Queue"=w289) -> ("error out"=w295:errorcluster)  [unwired: 9 in]
      n137 = call "Synchronize Caller Events.vi"("Singleton Module Admin in"=w290) -> ("error out"=w297:errorcluster)  [unwired: 9 in, 1 out]
      n138 = call "Module Name--constant.vi"() -> ("Module Name"=w293:string)  [unwired: 11 in]
      n139 = Format Into String(format string="An error occurred during initialization. %s is no longer running.", w293) -> (resulting string=w291:string)  [unwired: 2 in, 1 out]
      n140 = Merge Errors(w295, w297) -> (w298:errorcluster)
      n141 = call "Error Reported.vi"("Additional Information"=w291, "Error"=w298) -> ()  [unwired: 9 in, 1 out]
    }
  }
  n142 = Merge Errors(w14, w17) -> (w13:errorcluster)
  n143 = call "Close Module.vi"("error in"=w13, "Module Admin in"=w8) -> ("error out"=w15:errorcluster, "External Launch"=w2:bool, "Module Admin out"=w3:refnum<class "Delacor_lib_QMH_Module Admin.lvclass">)  [unwired: 7 in]
  n144 = Unregister For Events(event registration refnum=w7, error in=w15) -> (error out=w12:errorcluster)
  "error out" <- w12
  n145 = case "External Launch?" shown="True" w2 {
    tunnel: w12 -> [_ w299]
    frame False {
    }
    frame True {
      n146 = case shown="No Error" w299 {
        frame No Error {
          n147 = invoke on="Invoke Node" class="VI" method="FP.Close"() -> ()  [unwired: 3 in, 3 out]
        }
        frame Error {
          n148 = invoke on="Invoke Node" class="VI" method="FP.Open"("Activate"=TRUE ("Activate?")) -> ()  [unwired: 4 in, 5 out]
        }
      }
    }
  }
  n149 = local write "Module Admin"(w3) -> ()
